vi "search-variant.vi"(10 "Search":variant, 11 "Data (var) []":variant[](array[variant])) -> (2 "Index":i32)   [LabVIEW 2015, in "binary_search.lvlib"]
uses:
  binary_search.lvlib
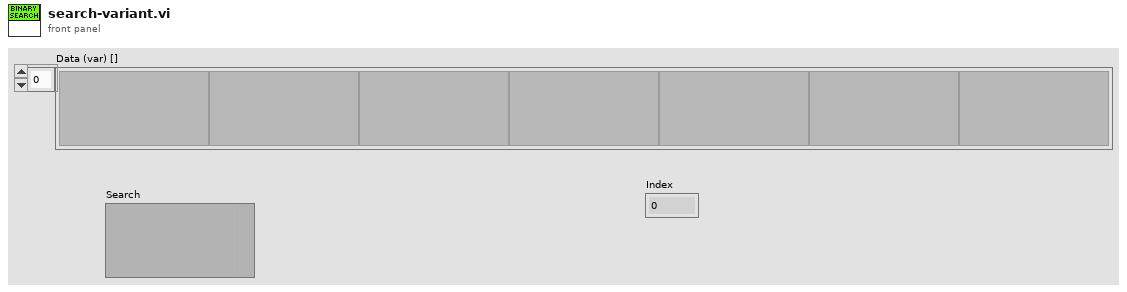
[diagram p1: front panel]
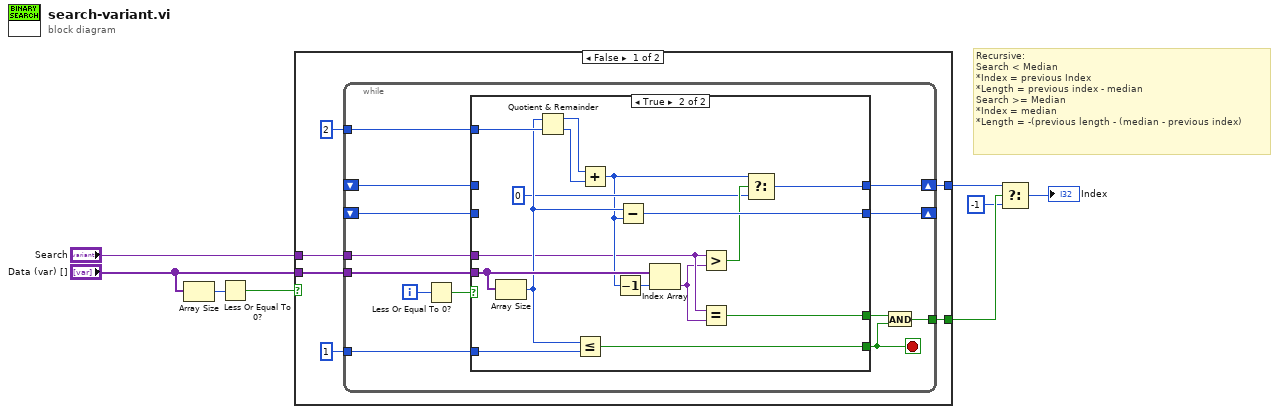
[diagram p0: block diagram]
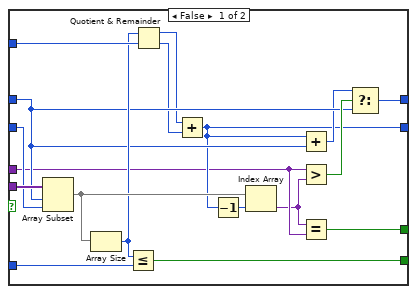
[diagram p2: hidden frame]
diagram:
  # "Recursive:\nSearch < Median\n*Index = previous Index\n*Length = previous index - median\nSearch >= Median\n*Index = median\n*Length = -(previous length - (median - previous index)"
  n1 = Array Size(array="Data (var) []") -> (size(s)=w6:i32)
  n2 = Less Or Equal To 0?(x=w6) -> (x <= 0?=w1:bool)
  n3 = case shown="False" w1 {
    tunnel: "Data (var) []" -> [w14 _]
    tunnel: "Search" -> [w13 _]
    tunnel: [w10 _] -> w5
    tunnel: [w9 _] -> w4
    frame False {
      n4 = while {
        tunnel: w14 -> [w25]
        tunnel: w13 -> [w27]
        shift-right: [w24] -> w9
        shift-left: _ -> [w26]
        shift-right: [w23] -> _
        shift-left: _ -> [w22]
        tunnel: 1 ("y") -> [w19]
        tunnel: 2 ("y") -> [w18]
        tunnel: [w15] -> w10
        i -> [w21]
        stop <- w16 stop-if-true
        n5 = Less Or Equal To 0?(x=w21) -> (x <= 0?=w20:bool)
        n6 = case shown="True" w20 {
          tunnel: w27 -> [w32 w49]
          tunnel: w26 -> [w36 _]
          tunnel: w25 -> [w45 w61]
          tunnel: [w41 w58] -> w24
          tunnel: [w33 w60] -> w23
          tunnel: w22 -> [w44 _]
          tunnel: [w30 w47] -> w16
          tunnel: w19 -> [w42 w57]
          tunnel: w18 -> [w39 w56]
          tunnel: [w28 w46] -> w17
          frame False {
            n7 = Array Subset(array=w45, index=w36, length=w44) -> (w43:variant[])
            n8 = Array Size(array=w43) -> (size(s)=w38:i32)
            n9 = Less Or Equal?(x=w38, y=w42) -> (x <= y?=w30:bool)
            n10 = Quotient & Remainder(x=w38, y=w39) -> (x-y*floor(x/y)=w34:i32, floor(x/y)=w29:i32)
            n11 = Add(x=w34, y=w29) -> (x+y=w33:i32)
            n12 = Decrement(x=w33) -> (x-1=w37:i32)
            n13 = Index Array(array=w43, index=w37) -> (element=w31:variant)
            n14 = Add(x=w33, y=w36) -> (x+y=w35:i32)
            n15 = Greater?(x=w32, y=w31) -> (0:w40:bool)
            n16 = Equal?(x=w31, y=w32) -> (x = y?=w28:bool)
            n17 = Select(t=w35, s=w40, f=w36) -> (s? t:f=w41:i32)
          }
          frame True {
            n18 = Array Size(array=w61) -> (size(s)=w55:i32)
            n19 = Quotient & Remainder(x=w55, y=w56) -> (x-y*floor(x/y)=w50:i32, floor(x/y)=w52:i32)
            n20 = Less Or Equal?(x=w55, y=w57) -> (x <= y?=w47:bool)
            n21 = Add(x=w50, y=w52) -> (x+y=w51:i32)
            n22 = Decrement(x=w51) -> (x-1=w53:i32)
            n23 = Subtract(x=w55, y=w51) -> (x-y=w60:i32)
            n24 = Index Array(array=w61, index=w53) -> (element=w48:variant)
            n25 = Greater?(x=w49, y=w48) -> (0:w59:bool)
            n26 = Equal?(x=w49, y=w48) -> (x = y?=w46:bool)
            n27 = Select(t=w51, s=w59, f=0) -> (s? t:f=w58:i32)
          }
        }
        n28 = And(x=w17, y=w16) -> (x .and. y?=w15:bool)
      }
    }
    frame True {
    }
  }
  n29 = Select(t=w4, s=w5, f=-1) -> (s? t:f=→"Index":i32)
